vi "MFC Flow.vi"(8 "error in (no error)":errorcluster, 10 "MFC Flow":waveform(dbl), 11 "MFC Flow in":refnum<class "MFC Flow.lvclass">) -> (0 "error out":errorcluster, 3 "MFC Flow out":refnum<class "MFC Flow.lvclass">)   [LabVIEW 2021, in "MFC Flow.lvlib" / "MFC Flow.lvclass"]
uses:
  MFC Flow.lvclass
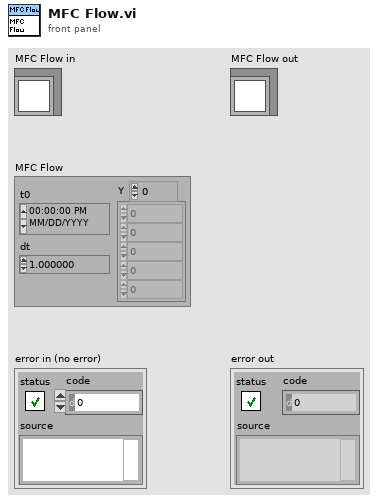
[diagram p1: front panel]
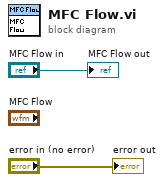
[diagram p0: block diagram]
diagram:
  "error out" <- "error in (no error)"
  "MFC Flow out" <- "MFC Flow in"
